vi "face reversecolumns.vi"(8 "error in (no error)":errorcluster, 11 "face in":T1) -> (0 "error out":errorcluster, 3 "face out":T1)   [LabVIEW 2011]
uses:
  Typedef/face.ctl
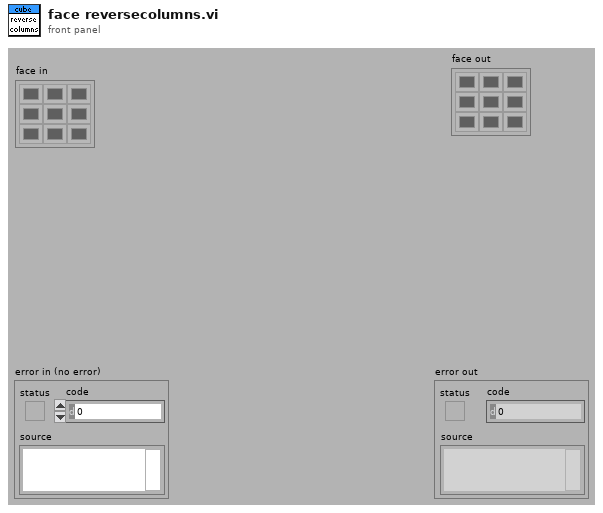
[diagram p1: front panel]
types:
  T1 = typedef "face.ctl" = u32[][]
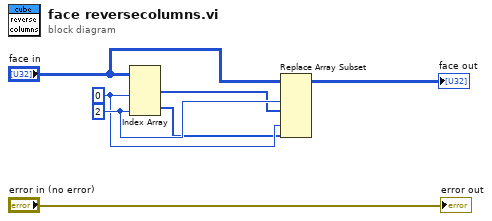
[diagram p0: block diagram]
diagram:
  w5 = 2 ("index (col)")
  w3 = 0 ("disabled index (col)")
  n1 = Index Array(array="face in", index (col) #1=w3, index (col) #2=w5) -> (element #1=w4:u32[], element #2=w2:u32[])  [unwired: 2 in]
  n2 = Replace Array Subset(array="face in", new element #1=w4, index (col) #1=w5, new element #2=w2, index (col) #2=w3) -> (→"face out":T1)  [unwired: 2 in]
  "error out" <- "error in (no error)"
